vi "Stop Core.vi"(10 "final error code":i32, 11 "Sensor in":refnum<class "Sensor.lvclass">) -> (3 "Sensor out":refnum<class "Sensor.lvclass">)   [LabVIEW 2016, in "Sensor.lvlib" / "Sensor.lvclass"]
doc: "In addition to the following, this method also sends a message to the monitor to notify it that the actor has stopped execution.\n\n(<B>Filename</B>: Actor Framework.lvlib:Actor.lvclass:Stop Core.vi)\n\nDefines what the actor does before it stops. Use the <B>final error code</B> input to determine whether the actor shut down in response to an error.\n\nBy default, this method does nothing. A descendant class may override it to define behavior, such as shutting down any processes the actor initiated in its override of the Actor Core method.\n\nCopyright: MGI\nAuthored by: Derek Trepanier"
uses:
  Sensor.lvclass
  Sensor.lvclass/Sensor.ctl
  Actor Monitor/Actor/Monitored Actor.lvclass
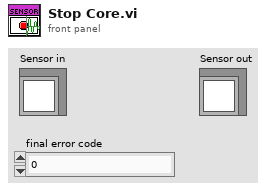
[diagram p1: front panel]
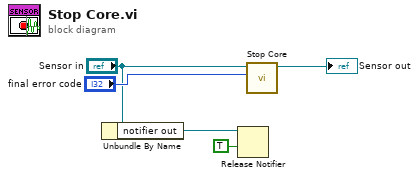
[diagram p0: block diagram]
diagram:
  n1 = Unbundle By Name("Sensor in") -> ("notifier out"=w2:refnum<notifier>)
  n2 = Release Notifier(notifier=w2, force destroy? (F)=TRUE) -> ()  [unwired: 1 in, 3 out]
  n3 = call-parent "Stop Core.vi"("final error code"="final error code", "Monitored Actor in"="Sensor in") -> ("Monitored Actor out"=→"Sensor out":refnum<class "Sensor.lvclass">)  [unwired: 9 in]
